vi "fgv_remote_udp_img.vi"(7 "cmd":enum16{"ini", "read", "write", "close"}(ring), 8 "error in":errorcluster) -> (0 "error out":errorcluster)   [LabVIEW 2019]
panel:
  out "LiDAR Image Gray":T1(plugin-control)
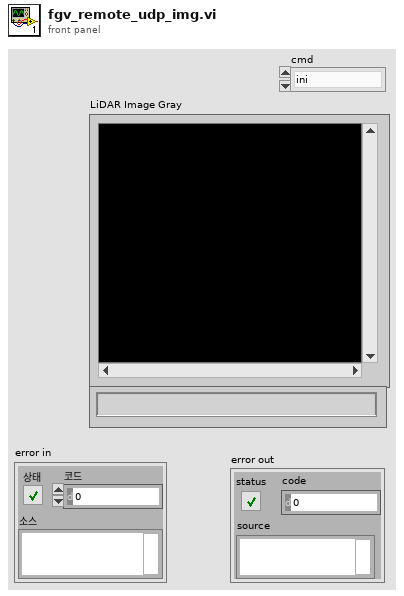
[diagram p1: front panel]
types:
  T1 = typedef "IMAQ Image.ctl" = refnum<image>
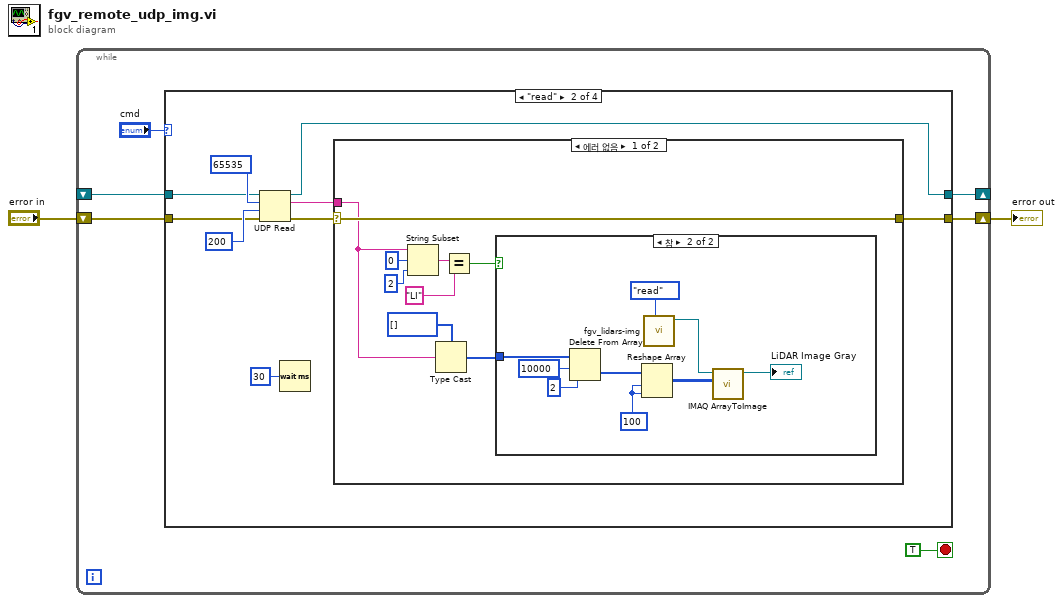
[diagram p0: block diagram]
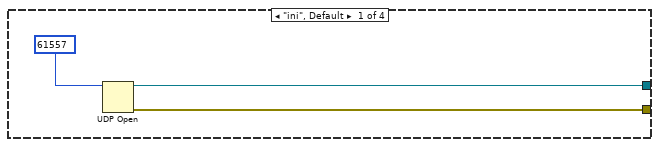
[diagram p2: hidden frame]
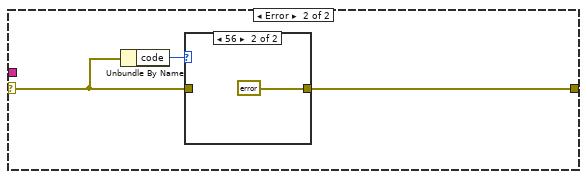
[diagram p4: hidden frame]
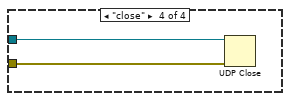
[diagram p7: hidden frame]
diagram:
  n1 = while {
    shift-right: [w5] -> _
    shift-left: _ -> [w4]
    shift-right: [w6] -> w2
    shift-left: "error in" -> [w3]
    stop <- TRUE stop-if-true
    n2 = case shown="\"read\"" "cmd" {
      tunnel: [w10 w12 w44 _] -> w6
      tunnel: [w9 w13 w45 _] -> w5
      tunnel: w4 -> [_ w15 w45 w47]
      tunnel: w3 -> [_ w14 w44 w46]
      frame "ini", Default {
        n3 = UDP Open(11:u16 61557 ("port")) -> (port=w9:refnum<k16>, 0:w10:errorcluster)  [unwired: 4 in, 1 out]
      }
      frame "read" {
        n4 = UDP Read(connection ID=w15, max size (548)=65535, timeout ms (25000)=200, 8:w14) -> (data out=w20:string, error out=w17:errorcluster, 3:w13:refnum<k16>)  [unwired: 2 out]
        n5 = Wait (ms)(milliseconds to wait=u32 30) -> ()  [unwired: 1 out]
        n6 = case shown="에러 없음" w17 {
          selector: w17 -> [w28 w41]
          tunnel: w20 -> [w23 _]
          tunnel: [w28 w39] -> w12
          frame No Error {
            n7 = String Subset(string=w23, offset (0)=0, length (rest)=2 ("length (rest)")) -> (substring=w25:string)
            n8 = Type Cast(type=u8[] [], x=w23) -> (*(type *) &x=w21:u8[])
            n9 = Equal?(x=w25, y="LI") -> (x = y?=w22:bool)
            n10 = case shown="참" w22 {
              tunnel: w21 -> [_ w38]
              frame False {
              }
              frame True {
                w36 = 100 ("dimension size")
                n11 = Delete From Array(array=w38, length=10000, index=2) -> (deleted portion=w32:u8[])  [unwired: 1 out]
                n12 = Reshape Array(w32, w36, w36) -> (w35:u8[][])
                n13 = call "fgv_lidars-img.vi"("cmd"=enum16{"create", "read", "close"}."read") -> ("New Image"=w30:T1)  [unwired: 10 in]
                n14 = call "IMAQ ArrayToImage"("Image Pixels (U8)"=w35, "Image"=w30) -> ("Image Out"=→"LiDAR Image Gray":T1)  [unwired: 8 in, 1 out]
              }
            }
          }
          frame Error {
            n15 = Unbundle By Name(w41) -> ("code"=w40:i32)
            n16 = case shown="56" w40 {
              tunnel: w41 -> [w42 _]
              tunnel: [w42 errorcluster {"status"=FALSE, "code"=0, "source"=""} ("error IO")] -> w39
              frame 0, Default {
              }
              frame 56 {
              }
            }
          }
        }
      }
      frame "write" {
      }
      frame "close" {
        n17 = UDP Close(connection ID=w47, 8:w46) -> ()  [unwired: 2 out]
      }
    }
  }
  "error out" <- w2
